vi "SetDigitalOutputs.vi"() -> ()   [LabVIEW 2020, in "HandsOnPi2040.lvlib"]
uses:
  <instrlib>/HandsOnPi2040/HandsOnPi2040.lvlib
  <instrlib>/HandsOnPi2040/Public/AOs.ctl
  <instrlib>/HandsOnPi2040/Public/DigIns.ctl
  <instrlib>/HandsOnPi2040/Public/AnaIns.ctl
  <instrlib>/HandsOnPi2040/Public/DigOuts.ctl
panel:
  out "LoopIndex":i32
  out "Firmware Version":string
  out "IDN":string
  in  "Digital Output":T1(ring)=enum."DO1"
  in  "DOBEEP":bool
  in  "DO4":bool
  in  "DO3":bool
  in  "DO2":bool
  in  "ANOutData":dbl[](array[numeric])
  in  "Analog Output 2":T2=enum."AO1" caption="AnOut Channel"
  in  "WriteAnOut":bool
  out "AnInValue":dbl(graph)
  in  "Analog Inputs":T3=enum."AI1"
  out "DIStatus":bool
  in  "Digital Inputs":T4=enum."DI1"
  out "AnOutValues":dbl[](graph)
  in  "Analog Output":T2=enum."AO1"
  out "DOStatus":bool
  in  "DO1":bool
  in  "VISA resource name":refnum<visa-resource-name>="TCPIP0::192.168.10.207::6430::SOCKET"
  out "error out":errorcluster
  in  "stop":bool
  # "READ"
  # "WRITE"
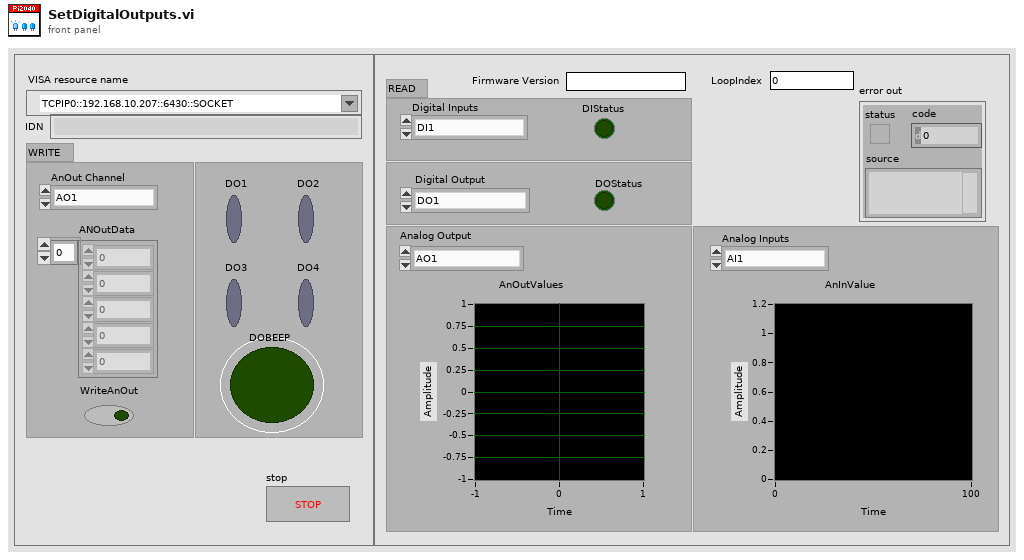
[diagram p1: front panel]
types:
  T1 = enum16{"No DO - Error", "DO1", "DO2", "DO3", "DO4", "BEEP"}
  T2 = typedef "HandsOnPi2040.lvlib/AOs.ctl" = enum16{"No AO - Error", "AO1"}
  T3 = typedef "HandsOnPi2040.lvlib/AnaIns.ctl" = enum16{"No AI - Error", "AI1", "AI2"}
  T4 = typedef "HandsOnPi2040.lvlib/DigIns.ctl" = enum16{"No DI - Error", "DI1", "DI2", "DI3", "DI4"}
  T5 = typedef "HandsOnPi2040.lvlib/DigOuts.ctl" = enum16{"No DO - Error", "DO1", "DO2", "DO3", "DO4", "BEEP"}
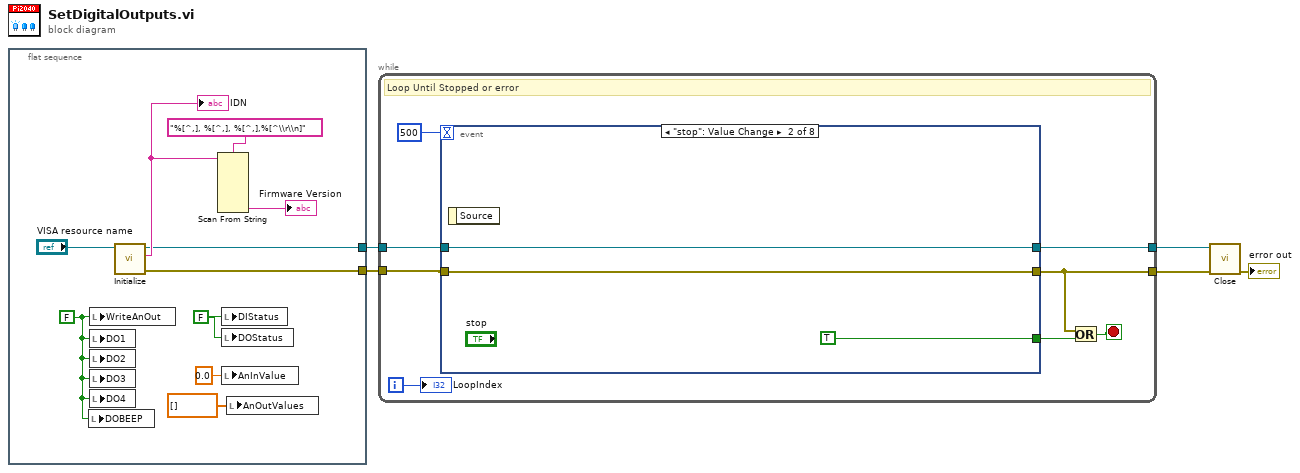
[diagram p0: block diagram]
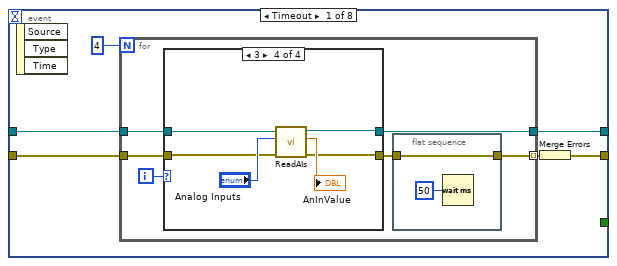
[diagram p2: hidden frame]
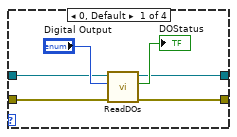
[diagram p3: hidden frame]
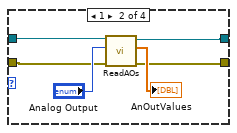
[diagram p4: hidden frame]
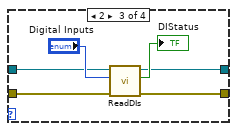
[diagram p5: hidden frame]
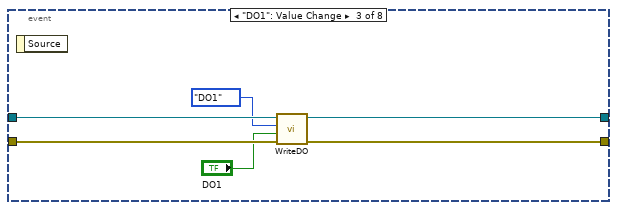
[diagram p6: hidden frame]
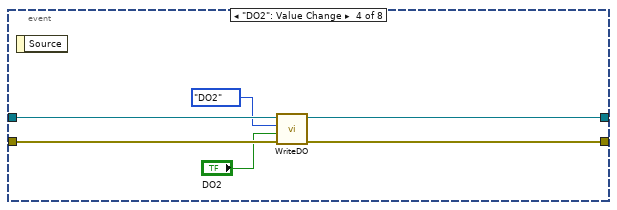
[diagram p7: hidden frame]
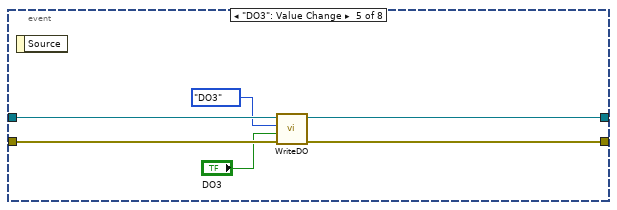
[diagram p8: hidden frame]
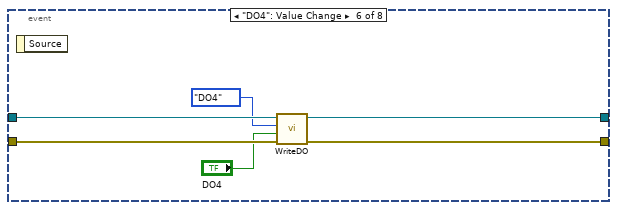
[diagram p9: hidden frame]
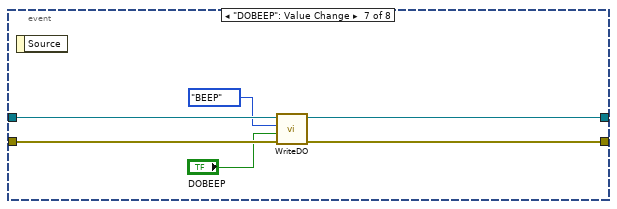
[diagram p10: hidden frame]
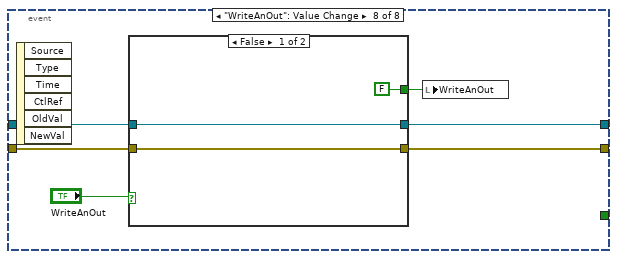
[diagram p11: hidden frame]
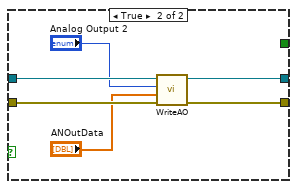
[diagram p12: hidden frame]
diagram:
  n1 = flat-sequence {
    tunnel: [w12] -> w2
    tunnel: [w11] -> w1
    frame #0 {
      w8 = FALSE ("WriteAnOut")
      w9 = FALSE ("WriteAnOut")
      n2 = local write "DOBEEP"(w9) -> ()
      n3 = local write "WriteAnOut"(w9) -> ()
      n4 = local write "DO1"(w9) -> ()
      n5 = local write "DO2"(w9) -> ()
      n6 = local write "DO3"(w9) -> ()
      n7 = local write "DO4"(w9) -> ()
      n8 = call <instrlib>:"Initialize.vi"("VISA resource name"="VISA resource name") -> ("error out"=w11:errorcluster, "IDN"=w13:string, "VISA resource name out"=w12:refnum<visa-resource-name>)  [unwired: 8 in]
      "IDN" <- w13
      n9 = Scan From String(format string="%[^,], %[^,], %[^,],%[^\\r\\n]", input string=w13) -> (output 4=→"Firmware Version":string)  [unwired: 9 in, 3 out]
      n10 = local write "DIStatus"(w8) -> ()
      n11 = local write "DOStatus"(w8) -> ()
      n12 = local write "AnInValue"(0.0 ("AnInValue")) -> ()
      n13 = local write "AnOutValues"(dbl[] [] ("AnOutValues")) -> ()
    }
  }
  n14 = while {
    tunnel: [w18] -> w5
    tunnel: w2 -> [w23]
    tunnel: [w22] -> w3
    tunnel: w1 -> [w20]
    i -> [w19]
    stop <- w16 stop-if-true
    # "Loop Until Stopped or error"
    n15 = event shown="[1] \"stop\": Value Change" {
      selector: _ -> [_ _ _ _ _ _ _ _]
      dyn-events: _ -> [_ _ _ _ _ _ _ _]
      timeout: 500 -> [_ _ _ _ _ _ _ _]
      tunnel: [_ TRUE _ _ _ _ _ _] -> w17
      tunnel: [w27 w62 w70 w76 w82 w88 w94 w100] -> w18
      tunnel: w20 -> [w29 w62 w69 w75 w81 w87 w93 w98]
      tunnel: w23 -> [w26 w63 w68 w74 w80 w86 w92 w97]
      tunnel: [w25 w63 w67 w73 w79 w85 w91 w99] -> w22
      event Timeout {
        n16 = event-data() -> ()  [unwired: 1 in, 3 out]
        n17 = for {
          N: 4 -> [_]
          tunnel: w29 -> [w34]
          tunnel: [w30] -> w28 mode=indexing
          tunnel: w26 -> [w33]
          tunnel: [w32] -> w25
          i -> [w35]
          n18 = case shown="3" w35 {
            tunnel: w34 -> [w41 w46 w52 w58]
            tunnel: [w40 w44 w50 w56] -> w31
            tunnel: w33 -> [w39 w47 w53 w59]
            tunnel: [w38 w45 w51 w57] -> w32
            frame 0, Default {
              n19 = call <instrlib>:"ReadDOs.vi"("error in (no error)"=w41, "Output"="Digital Output", "VISA resource name"=w39) -> ("error out"=w40:errorcluster, "DOStatus"=→"DOStatus":bool, "VISA resource name out"=w38:refnum<visa-resource-name>)  [unwired: 6 in]
            }
            frame 1 {
              n20 = call <instrlib>:"ReadAOs.vi"("error in (no error)"=w46, "Analog Output"="Analog Output", "VISA resource name"=w47) -> ("error out"=w44:errorcluster, "AnOutValues"=→"AnOutValues":dbl[], "VISA resource name out"=w45:refnum<visa-resource-name>)  [unwired: 6 in]
            }
            frame 2 {
              n21 = call <instrlib>:"ReadDIs.vi"("error in (no error)"=w52, "Digital Inputs"="Digital Inputs", "VISA resource name"=w53) -> ("error out"=w50:errorcluster, "DIStatus"=→"DIStatus":bool, "VISA resource name out"=w51:refnum<visa-resource-name>)  [unwired: 6 in]
            }
            frame 3 {
              n22 = call <instrlib>:"ReadAIs.vi"("error in (no error)"=w58, "Analog Inputs"="Analog Inputs", "VISA resource name"=w59) -> ("error out"=w56:errorcluster, "AnInValue"=→"AnInValue":dbl, "VISA resource name out"=w57:refnum<visa-resource-name>)  [unwired: 6 in]
            }
          }
          n23 = flat-sequence {
            tunnel: w31 -> [w37]
            tunnel: [w37] -> w30
            frame #0 {
              n24 = Wait (ms)(milliseconds to wait=u32 50) -> ()  [unwired: 1 out]
            }
          }
        }
        n25 = Merge Errors(w28) -> (w27:errorcluster)
      }
      event "stop": Value Change {
        n26 = event-data() -> ()  [unwired: 1 in, 1 out]
      }
      event "DO1": Value Change {
        n27 = event-data() -> ()  [unwired: 1 in, 1 out]
        n28 = call <instrlib>:"WriteDO.vi"("error in (no error)"=w69, "DO Value (True)"="DO1", "Output"=DigOuts."DO1" ("Write Digital Output"), "VISA resource name"=w68) -> ("error out"=w70:errorcluster, "VISA resource name out"=w67:refnum<visa-resource-name>)  [unwired: 6 in]
      }
      event "DO2": Value Change {
        n29 = event-data() -> ()  [unwired: 1 in, 1 out]
        n30 = call <instrlib>:"WriteDO.vi"("error in (no error)"=w75, "DO Value (True)"="DO2", "Output"=DigOuts."DO2" ("Write Digital Output"), "VISA resource name"=w74) -> ("error out"=w76:errorcluster, "VISA resource name out"=w73:refnum<visa-resource-name>)  [unwired: 6 in]
      }
      event "DO3": Value Change {
        n31 = event-data() -> ()  [unwired: 1 in, 1 out]
        n32 = call <instrlib>:"WriteDO.vi"("error in (no error)"=w81, "DO Value (True)"="DO3", "Output"=DigOuts."DO3" ("Write Digital Output"), "VISA resource name"=w80) -> ("error out"=w82:errorcluster, "VISA resource name out"=w79:refnum<visa-resource-name>)  [unwired: 6 in]
      }
      event "DO4": Value Change {
        n33 = event-data() -> ()  [unwired: 1 in, 1 out]
        n34 = call <instrlib>:"WriteDO.vi"("error in (no error)"=w87, "DO Value (True)"="DO4", "Output"=DigOuts."DO4" ("Write Digital Output"), "VISA resource name"=w86) -> ("error out"=w88:errorcluster, "VISA resource name out"=w85:refnum<visa-resource-name>)  [unwired: 6 in]
      }
      event "DOBEEP": Value Change {
        n35 = event-data() -> ()  [unwired: 1 in, 1 out]
        n36 = call <instrlib>:"WriteDO.vi"("error in (no error)"=w93, "DO Value (True)"="DOBEEP", "Output"=DigOuts."BEEP" ("Write Digital Output"), "VISA resource name"=w92) -> ("error out"=w94:errorcluster, "VISA resource name out"=w91:refnum<visa-resource-name>)  [unwired: 6 in]
      }
      event "WriteAnOut": Value Change {
        n37 = event-data() -> ()  [unwired: 1 in, 6 out]
        n38 = case shown="False" "WriteAnOut" {
          tunnel: [w102 w109] -> w100
          tunnel: [w103 w108] -> w99
          tunnel: w98 -> [w102 w107]
          tunnel: w97 -> [w103 w106]
          tunnel: [FALSE _] -> w95
          frame False {
          }
          frame True {
            n39 = call <instrlib>:"WriteAO.vi"("error in (no error)"=w107, "Array"="ANOutData", "Analog Output"="Analog Output 2", "VISA resource name"=w106) -> ("error out"=w109:errorcluster, "VISA resource name out"=w108:refnum<visa-resource-name>)  [unwired: 6 in]
          }
        }
        n40 = local write "WriteAnOut"(w95) -> ()
      }
    }
    n41 = Or(x=w18, y=w17) -> (x .or. y?=w16:bool)
    "LoopIndex" <- w19
  }
  n42 = call <instrlib>:"Close.vi"("error in (no error)"=w5, "VISA resource name"=w3) -> ("error out"=→"error out":errorcluster)  [unwired: 9 in]
